vi "Event Is Nested.vi"(10 "Alias":string, 11 "Queue jettl in":refnum<class "Queue jettl.lvclass">) -> (2 "Event Is Nested?":bool)   [LabVIEW 2021, in "jettl.lvlib" / "Queue jettl.lvclass"]
uses:
  Queue jettl.lvclass
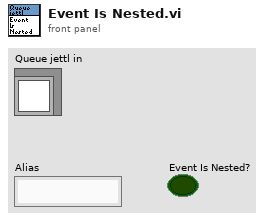
[diagram p1: front panel]
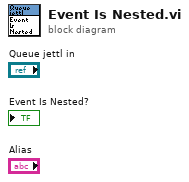
[diagram p0: block diagram]
diagram:
